vi "hmi_scriptbuttons.vi"(11 "UserData":T1) -> ()   [LabVIEW 2011]
uses:
  user_data.ctl
  user_buttons_dualaction.ctl
  user_buttons_360.ctl
  script/MutexMode.ctl
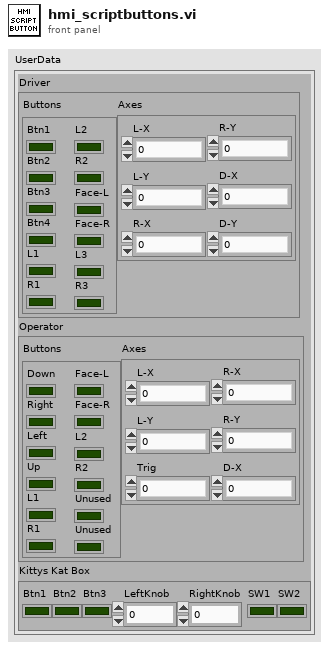
[diagram p1: front panel]
types:
  T1 = typedef "user_data.ctl" = cluster{"Driver":cluster{"Buttons":T2, "Axes":cluster{"L-X":dbl, "L-Y":dbl, "R-X":dbl, "R-Y":dbl, "D-X":dbl, "D-Y":dbl}}, "Operator":cluster{"Buttons":T3, "Axes":cluster{"L-X":dbl, "L-Y":dbl, "Trig":dbl, "R-X":dbl, "R-Y":dbl, "D-X":dbl}}, "Kittys Kat Box":cluster{"Btn1":bool, "Btn2":bool, "Btn3":bool, "LeftKnob":dbl, "RightKnob":dbl, "SW1":bool, "SW2":bool}}
  T2 = typedef "user_buttons_dualaction.ctl" = cluster{"Btn1":bool, "Btn2":bool, "Btn3":bool, "Btn4":bool, "L1":bool, "R1":bool, "L2":bool, "R2":bool, "Face-L":bool, "Face-R":bool, "L3":bool, "R3":bool}
  T3 = typedef "user_buttons_360.ctl" = cluster{"Down":bool, "Right":bool, "Left":bool, "Up":bool, "L1":bool, "R1":bool, "Face-L":bool, "Face-R":bool, "L2":bool, "R2":bool, "Unused":bool, "Unused":bool}
  T4 = typedef "MutexMode.ctl" = enum16{"Get Mode", "Request Execution", "Stop Execution", "Lock Autonomous", "Script Completed"}
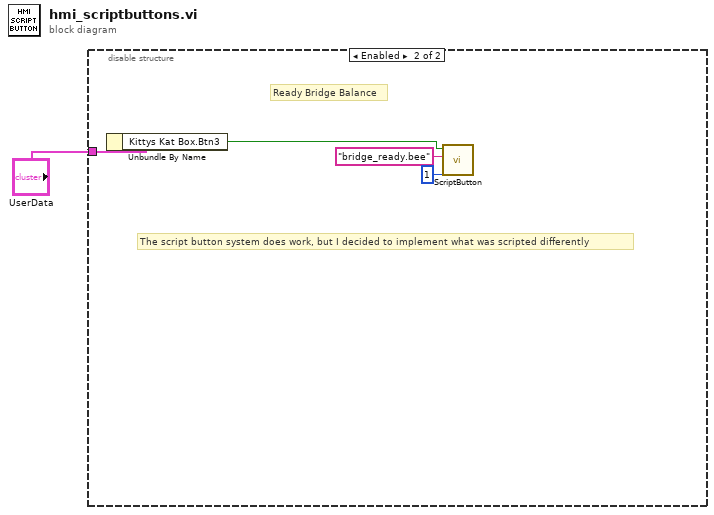
[diagram p0: block diagram]
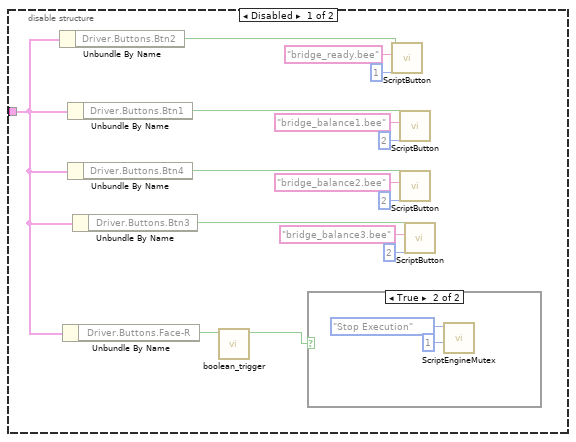
[diagram p2: hidden frame]
diagram:
  n1 = disable-structure shown="Enabled" {
    disable-tunnel: "UserData" -> [w2 w22]
    frame Disabled {
      n2 = Unbundle By Name(w2) -> ("Driver.Buttons.Btn2"=w5:bool)
      n3 = Unbundle By Name(w2) -> ("Driver.Buttons.Face-R"=w6:bool)
      n4 = Unbundle By Name(w2) -> ("Driver.Buttons.Btn1"=w16:bool)
      n5 = Unbundle By Name(w2) -> ("Driver.Buttons.Btn4"=w13:bool)
      n6 = Unbundle By Name(w2) -> ("Driver.Buttons.Btn3"=w10:bool)
      n7 = call "boolean_trigger.vi"("Input"=w6) -> ("Rising Edge"=w7:bool)  [unwired: 10 in]
      n8 = case shown="True" w7 {
        frame False {
        }
        frame True {
          n9 = call "ScriptEngineMutex.vi"("Priority"=u8 1, "Mutex Mode"=MutexMode."Stop Execution") -> ()  [unwired: 9 in, 1 out]
        }
      }
      n10 = call "ScriptButton.vi"("Priority"=u8 1, "Script Name"="bridge_ready.bee", "Button"=w5) -> ()  [unwired: 9 in]
      n11 = call "ScriptButton.vi"("Priority"=u8 2, "Script Name"="bridge_balance1.bee", "Button"=w16) -> ()  [unwired: 9 in]
      n12 = call "ScriptButton.vi"("Priority"=u8 2, "Script Name"="bridge_balance2.bee", "Button"=w13) -> ()  [unwired: 9 in]
      n13 = call "ScriptButton.vi"("Priority"=u8 2, "Script Name"="bridge_balance3.bee", "Button"=w10) -> ()  [unwired: 9 in]
    }
    frame Enabled {
      # "The script button system does work, but I decided to implement what was scripted differently"
      # "Ready Bridge Balance"
      n14 = Unbundle By Name(w22) -> ("Kittys Kat Box.Btn3"=w19:bool)
      n15 = call "ScriptButton.vi"("Priority"=u8 1, "Script Name"="bridge_ready.bee", "Button"=w19) -> ()  [unwired: 9 in]
    }
  }
